vi "SRV_PM_Create and Write Packet.vi"(0 "SRV ref":refnum<k5>, 1 "SRV IP Address":string, 5 "Command Type":string, 7 "Data String":string, 11 "error in (no error)":errorcluster) -> (4 "SRV ref out":refnum<k5>, 15 "error out":errorcluster)   [LabVIEW 2009]
doc: "Wire <B>either</B> SRV ref <B>or</B> SRV IP Address.\n\n\nAuthor: Mike Schultz"
panel:
  out "Data":u8[](array[numeric]) format="%.0x"
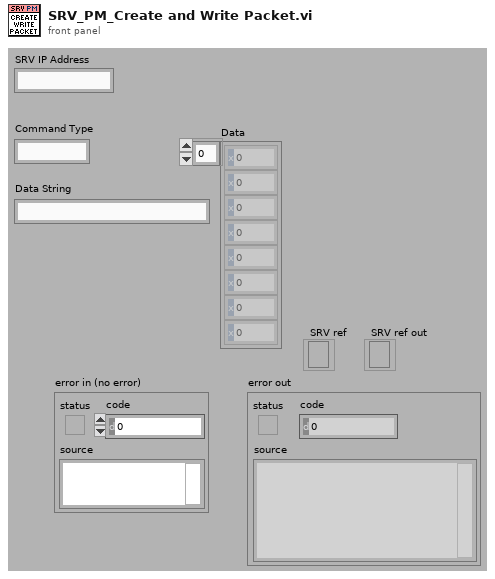
[diagram p1: front panel]
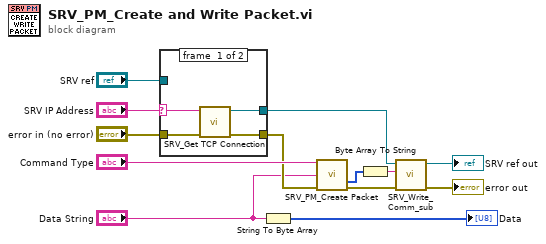
[diagram p0: block diagram]
diagram:
  n1 = case shown="Default" "SRV IP Address" {
    selector: "SRV IP Address" -> [w14 _]
    tunnel: [w17 w19] -> w6
    tunnel: "error in (no error)" -> [w16 w18]
    tunnel: [w15 w18] -> w4
    tunnel: "SRV ref" -> [_ w19]
    frame #0 {
      n2 = call "SRV_Get TCP Connection.vi"("error in (no error)"=w16, "IP address"=w14) -> ("error out"=w15:errorcluster, "connection ID"=w17:refnum<k5>)  [unwired: 8 in]
    }
    frame #1 {
    }
  }
  n3 = String To Byte Array(string="Data String") -> (unsigned byte array=→"Data":u8[])
  n4 = call "SRV_PM_Create Packet.vi"("Command Type"="Command Type", "Data String"="Data String", "error in (no error)"=w4) -> ("Packet"=w10:u8[], "error out"=w11:errorcluster)  [unwired: 11 in]
  n5 = Byte Array To String(unsigned byte array=w10) -> (string=w9:string)
  n6 = call "SRV_Write_Comm_sub.vi"("error in (no error)"=w11, "Command Sent"=w9, "SRV In"=w6) -> ("error out"=→"error out":errorcluster, "SRV Out"=→"SRV ref out":refnum<k5>)  [unwired: 6 in, 1 out]
